vi "TSM Relay Connect or Disconnect.vi"(0 "TSM context":T1, 5 "Relay Action":T2=21 items=["Open Relay"=20, "Close Relay"=21], 7 "Settling Time (s)":dbl=0.0001, 9 "Relays":tag[](array[tag]), 11 "error in":errorcluster) -> (4 "TSM context out":T1, 15 "error out":errorcluster)   [LabVIEW 2019]
uses:
  <vilib>/NI_TestStand_SemiconductorModule/NI_TestStand_Semiconductor_Module.lvlibp/PinMap/General/SemiconductorModuleContext.ctl
  <vilib>/NI_TestStand_SemiconductorModule/NI_TestStand_Semiconductor_Module.lvlibp/1abvi3w/instr.lib/niSwitch/niswitch.llb/niSwitch Relay Action.ctl
  Pin Map/TSM Relay.ctl
  <vilib>/NI_TestStand_SemiconductorModule/NI_TestStand_Semiconductor_Module.lvlibp/PinMap/Relay Driver/ControlRelay(s).vi
  <vilib>/NI_TestStand_SemiconductorModule/NI_TestStand_Semiconductor_Module.lvlibp/PinMap/Relay Driver/ControlRelaysSingleAction.vi
  <vilib>/Utility/High Resolution Polling Wait.vi
  <vilib>/NI_TestStand_SemiconductorModule/NI_TestStand_Semiconductor_Module.lvlibp
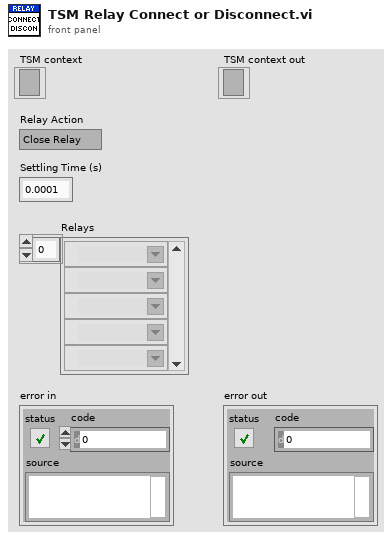
[diagram p1: front panel]
types:
  T1 = typedef "NI_TestStand_Semiconductor_Module.lvlibp/SemiconductorModuleContext.ctl" = refnum<k7>
  T2 = typedef "NI_TestStand_Semiconductor_Module.lvlibp/niSwitch Relay Action.ctl" = i32
  T3 = cluster{"Meas & Results":cluster{"Reserved":dbl[][]}}
  T4 = typedef "TSM Relay.ctl" = cluster{"TSM Context":T1, "Relays":tag[]}
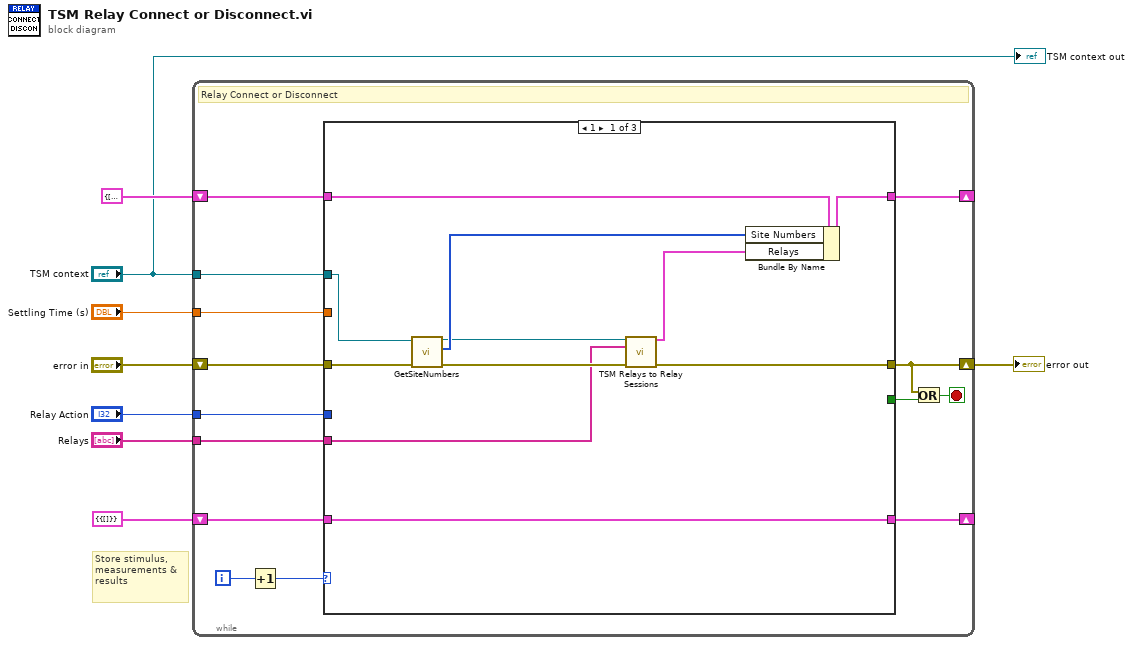
[diagram p0: block diagram]
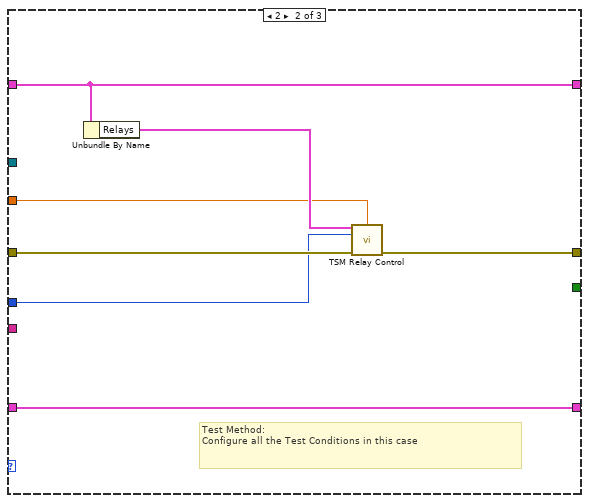
[diagram p2: hidden frame]
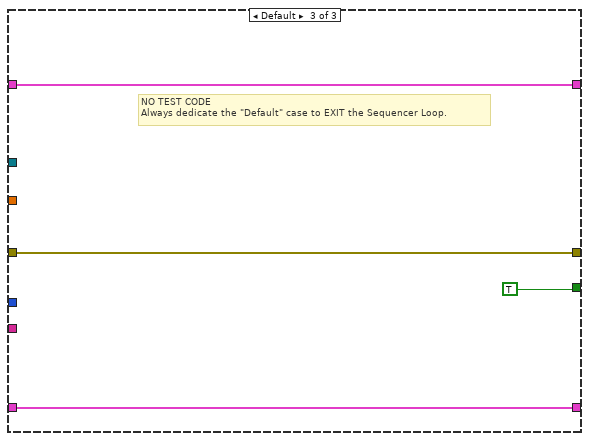
[diagram p3: hidden frame]
diagram:
  # "Store stimulus, measurements & results"
  n1 = while {
    shift-right: [w14] -> w8
    shift-left: "error in" -> [w21]
    tunnel: "TSM context" -> [w19]
    shift-right: [w16] -> _
    shift-left: cluster{"Site Numbers":i32[], "Relays":T4} {"Site Numbers"=[], "Relays"={"TSM Context"=refnum, "Relays"=[]}} -> [w17]
    shift-right: [w13] -> _
    shift-left: T3 {"Meas & Results"={"Reserved"=[]}} ("TCs") -> [w12]
    tunnel: "Relays" -> [w11]
    tunnel: "Relay Action" -> [w10]
    tunnel: "Settling Time (s)" -> [w9]
    i -> [w22]
    stop <- w15 stop-if-true
    # "Relay Connect or Disconnect"
    n2 = Increment(x=w22) -> (x+1=w20:i32)
    n3 = case shown="1" w20 {
      tunnel: [w26 w38 w43] -> w14
      tunnel: w21 -> [w33 w39 w43]
      tunnel: w19 -> [w28 _ _]
      tunnel: [_ _ TRUE] -> w18
      tunnel: w17 -> [w32 w37 w42]
      tunnel: [w31 w37 w42] -> w16
      tunnel: [w30 w40 w41] -> w13
      tunnel: w12 -> [w30 w40 w41]
      tunnel: w11 -> [w25 _ _]
      tunnel: w10 -> [_ w35 _]
      tunnel: w9 -> [_ w34 _]
      frame 1 {
        # "Get Instrument References\nDO NOT CHANGE IF NO ADDITIONAL PINS"
        n4 = call <vilib>:"GetSiteNumbers.vi"("error in (no error)"=w33, "Semiconductor Module Context"=w28) -> ("error out"=w27:errorcluster, "Site Numbers"=w29:i32[], "Semiconductor Module Context Out"=w23:T1)  [unwired: 6 in, 1 out]
        n5 = call "TSM Relays to Relay Sessions.vi"("TSM Context"=w23, "Relays"=w25, "error in (no error)"=w27) -> ("TSM Relay Out"=w24:T4, "error out"=w26:errorcluster)  [unwired: 11 in]
        n6 = Bundle By Name(cluster=w32, "Site Numbers"=w29, "Relays"=w24) -> (w31:cluster{"Site Numbers":i32[], "Relays":T4})
      }
      frame 2 {
        # "Test Method:\nConfigure all the Test Conditions in this case"
        # "Test Conditions and Instrument Settings"
        n7 = Unbundle By Name(w37) -> ("Relays"=w36:T4)
        n8 = call "TSM Relay Control.vi"("Relay TSM in"=w36, "Settling Time (s)"=w34, "Relay Action"=w35, "error in"=w39) -> ("error out"=w38:errorcluster)  [unwired: 11 in]
      }
      frame Default {
        # "NO TEST CODE\nAlways dedicate the \"Default\" case to EXIT the Sequencer Loop."
        # "Exit Loop"
      }
    }
    n9 = Or(x=w14, y=w18) -> (x .or. y?=w15:bool)
  }
  "error out" <- w8
  "TSM context out" <- "TSM context"
